vi "Shutdown IO.vi"(8 "error in":errorcluster, 11 "CRDS in":refnum<class "CRDS.lvclass">) -> (0 "error out":errorcluster, 3 "CRDS out":refnum<class "CRDS.lvclass">)   [LabVIEW 2011, in "CRDS.lvclass"]
uses:
  CRDS.lvclass
  Program Files (x86)/National Instruments/LabVIEW 2011/resource/objmgr/daqmx.rc
  Reusable/Serial IO/Base/Serial IO.lvclass
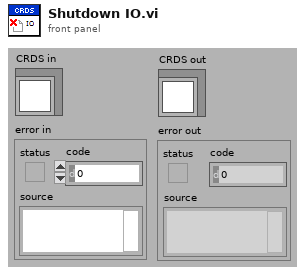
[diagram p1: front panel]
types:
  T1 = cluster{"YAG Ctr":refnum<k21>, "Diode Ctr":refnum<k21>, "Gated Ctr":refnum<k21>, "LF AI":refnum<k21>, "HF AI":refnum<k21>, "valveIn":refnum<k21>, "valveOut":refnum<k21>}
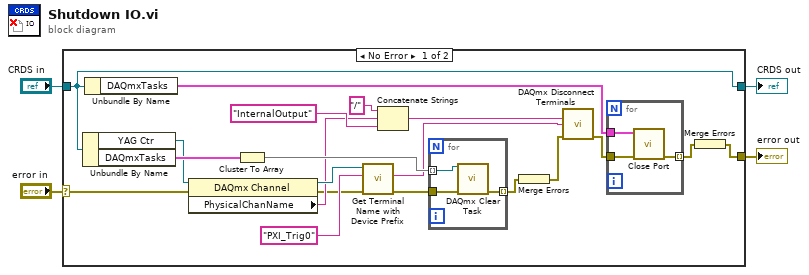
[diagram p0: block diagram]
diagram:
  n1 = case shown="No Error" "error in" {
    selector: "error in" -> [w8 w32]
    tunnel: [w12 w32] -> w3
    tunnel: [w16 w31] -> w1
    tunnel: "CRDS in" -> [w16 w31]
    frame No Error {
      n2 = Unbundle By Name(w16) -> ("YAG Ctr"=w9:refnum<k21>, "DAQmxTasks"=w23:T1)
      n3 = Unbundle By Name(w16) -> ("DAQmxTasks"=w15:T1)
      n4 = property class="DAQmx Channel"(reference=w9, error in=w8) -> (reference out=w11:refnum<k21>, error out=w7:errorcluster, "PhysicalChanName"=w10:tag)
      n5 = Cluster To Array(cluster=w23) -> (array=w24:refnum<k21>[])
      n6 = call "Get Terminal Name with Device Prefix.vi"("error in (no error)"=w7, "Local Terminal Name"="PXI_Trig0", "task/channels in"=w11) -> ("error out"=w6:errorcluster, "Terminal Name with Device Prefix"=w19:tag)  [unwired: 6 in, 1 out]
      n7 = Concatenate Strings("/", w10, "InternalOutput" ("string")) -> (w18:string)
      n8 = for {
        tunnel: w24 -> [w30] mode=indexing
        tunnel: [w29] -> w17 mode=indexing
        tunnel: w6 -> [w28]
        n9 = call <vilib>:"DAQmx Clear Task.vi"("task in"=w30, "error in"=w28) -> ("error out"=w29:errorcluster)  [unwired: 13 in]
      }
      n10 = Merge Errors(w17) -> (w5:errorcluster)
      n11 = call <vilib>:"DAQmx Disconnect Terminals.vi"("source terminal"=w18, "destination terminal"=w19, "error in"=w5) -> ("error out"=w14:errorcluster)  [unwired: 12 in]
      n12 = for {
        tunnel: w15 -> [w27]
        tunnel: w14 -> [w26]
        tunnel: [w25] -> w13 mode=indexing
        n13 = call-dynamic "Close Port.vi"("error in (no error)"=w26, "Serial IO in"=w27) -> ("error out"=w25:errorcluster)  [unwired: 8 in, 1 out]
      }
      n14 = Merge Errors(w13) -> (w12:errorcluster)
    }
    frame Error {
    }
  }
  "error out" <- w3
  "CRDS out" <- w1
